vi "TagDB Refmgr-Register.vi"(8 "error in (no error)":errorcluster, 9 "ViName":string, 10 "VI Refnum":refnum<vi>, 11 "TagDB in":T1) -> (0 "error out":errorcluster, 2 "VI Refnum (dup)":refnum<vi>, 3 "TagDB out":T1)   [LabVIEW 2017, in "TagDB RefManager.lvlib"]
uses:
  TagDB RefManager.lvlib
  <userlib>/_NEVSTOP/TagDB/Typedef/TagDB.ctl
  _Support/Refnum Operation/VI/Caller's VI Reference.vi
  _Support/Refnum Operation/VI/VIName.vi
  <userlib>/_NEVSTOP/TagDB/TagDB.lvlib
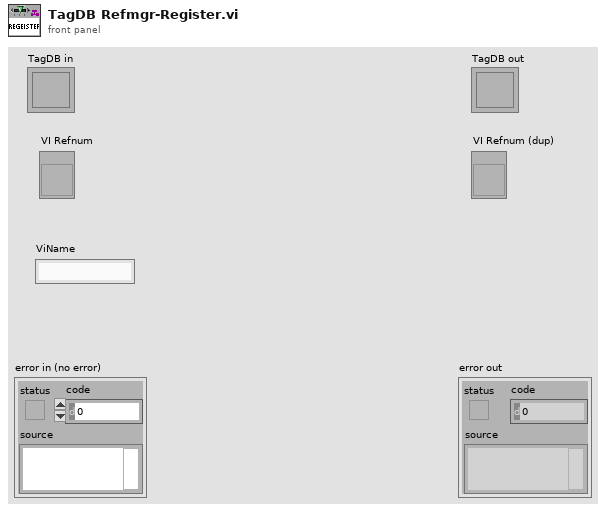
[diagram p1: front panel]
types:
  T1 = typedef "TagDB.lvlib/TagDB.ctl" = refnum<k1>
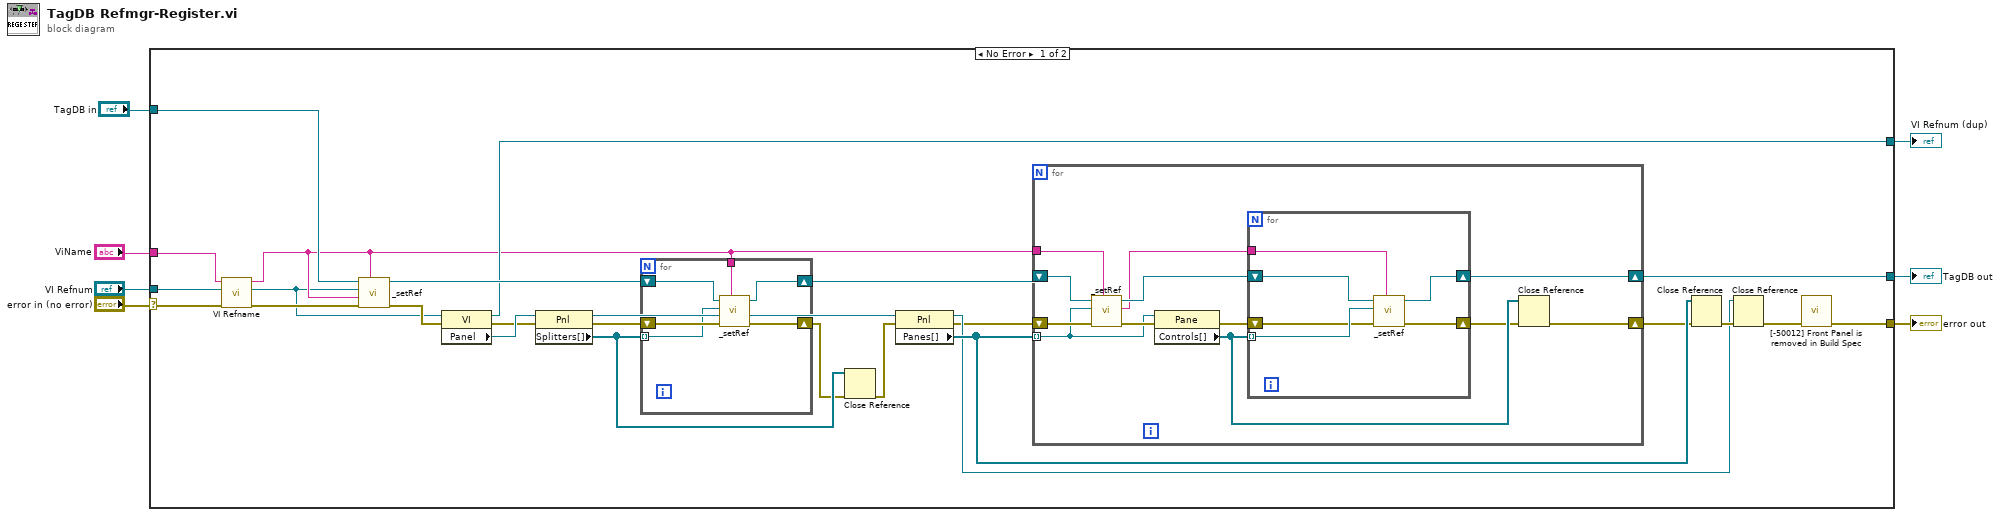
[diagram p0: block diagram]
diagram:
  n1 = case shown="No Error" "error in (no error)" {
    selector: "error in (no error)" -> [w14 w60]
    tunnel: [w12 w60] -> w6
    tunnel: [w32 w59] -> w4
    tunnel: "TagDB in" -> [w17 w59]
    tunnel: "VI Refnum" -> [w10 w58]
    tunnel: "ViName" -> [w11 _]
    tunnel: [w15 w58] -> w1
    frame No Error {
      n2 = call "VI Refname.vi"("error in (no error)"=w14, "VI in"=w10, "ViName"=w11) -> ("error out"=w19:errorcluster, "VI out"=w8:refnum<vi>, "Name"=w9:string)  [unwired: 6 in]
      n3 = call "_setRef.vi"("parentURL"=w9, "error in (no error)"=w19, "Name"=w9, "Refnum"=w8, "TagDB in"=w17) -> ("error out"=w18:errorcluster, "TagDB out"=w16:T1)  [unwired: 4 in, 1 out]
      n4 = property class="VI"(reference=w8, error in=w18) -> (reference out=w15:refnum<vi>, error out=w26:errorcluster, "Panel"=w27:refnum<vi>)
      n5 = property class="Pnl"(reference=w27, error in=w26) -> (reference out=w25:refnum<vi>, error out=w23:errorcluster, "Splitters[]"=w22:refnum<vi>[])
      n6 = for {
        shift-right: [w37] -> w24
        shift-left: w16 -> [w38]
        tunnel: w22 -> [w35] mode=indexing
        shift-right: [w36] -> w21
        shift-left: w23 -> [w39]
        tunnel: w9 -> [w34]
        n7 = call "_setRef.vi"("parentURL"=w34, "error in (no error)"=w39, "Refnum"=w35, "TagDB in"=w38) -> ("error out"=w36:errorcluster, "TagDB out"=w37:T1)  [unwired: 5 in, 1 out]
      }
      n8 = Close Reference(reference=w22, error in (no error)=w21) -> (error out=w20:errorcluster)
      n9 = property class="Pnl"(reference=w25, error in=w20) -> (reference out=w29:refnum<vi>, error out=w28:errorcluster, "Panes[]"=w33:refnum<vi>[])
      n10 = for {
        tunnel: w33 -> [w42] mode=indexing
        shift-right: [w50] -> w32
        shift-left: w24 -> [w44]
        shift-right: [w47] -> w31
        shift-left: w28 -> [w46]
        tunnel: w9 -> [w41]
        n11 = call "_setRef.vi"("parentURL"=w41, "error in (no error)"=w46, "Refnum"=w42, "TagDB in"=w44) -> ("error out"=w45:errorcluster, "URL"=w40:string, "TagDB out"=w43:T1)  [unwired: 5 in]
        n12 = property class="Pane"(reference=w42, error in=w45) -> (error out=w49:errorcluster, "Controls[]"=w51:refnum<vi>[])  [unwired: 1 out]
        n13 = for {
          tunnel: w51 -> [w54] mode=indexing
          shift-right: [w56] -> w50
          shift-left: w43 -> [w57]
          shift-right: [w55] -> w48
          shift-left: w49 -> [w53]
          tunnel: w40 -> [w52]
          n14 = call "_setRef.vi"("parentURL"=w52, "error in (no error)"=w53, "Refnum"=w54, "TagDB in"=w57) -> ("error out"=w55:errorcluster, "TagDB out"=w56:T1)  [unwired: 5 in, 1 out]
        }
        n15 = Close Reference(reference=w51, error in (no error)=w48) -> (error out=w47:errorcluster)
      }
      n16 = Close Reference(reference=w33, error in (no error)=w31) -> (error out=w30:errorcluster)
      n17 = Close Reference(reference=w29, error in (no error)=w30) -> (error out=w13:errorcluster)
      n18 = call "[-50012] Front Panel is removed in Build Spec.vi"("error in (no error)"=w13) -> ("error out"=w12:errorcluster)  [unwired: 10 in]
    }
    frame Error {
    }
  }
  "error out" <- w6
  "TagDB out" <- w4
  "VI Refnum (dup)" <- w1
